vi "GetOuterLoopDataField.vi"(10 "Telemetry Data":string, 11 "Cluster in":refnum<vi>) -> (3 "Array":string[](array[string]))   [LabVIEW 2016]
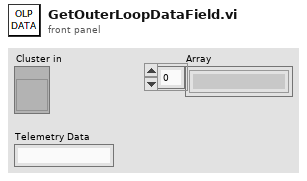
[diagram p1: front panel]
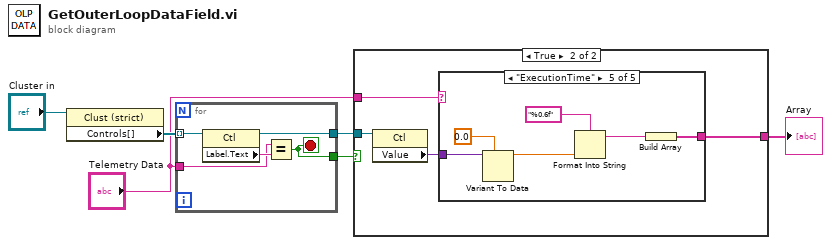
[diagram p0: block diagram]
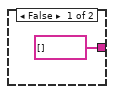
[diagram p2: hidden frame]
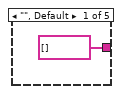
[diagram p3: hidden frame]
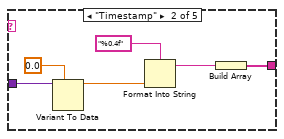
[diagram p4: hidden frame]
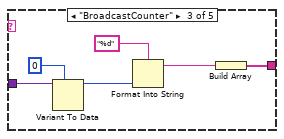
[diagram p5: hidden frame]
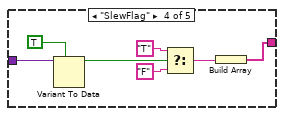
[diagram p6: hidden frame]
diagram:
  n1 = property on="Property Node" class="Clust (strict)"(reference="Cluster in") -> ("Controls[]"=w5:refnum<vi>[])  [unwired: 1 in, 2 out]
  n2 = for {
    tunnel: w5 -> [w11] mode=indexing
    tunnel: [w10] -> w2
    tunnel: "Telemetry Data" -> [w8]
    tunnel: [w7] -> w1
    stop <- w7 stop-if-true
    n3 = property on="Property Node" class="Ctl"(reference=w11) -> (reference out=w10:refnum<vi>, "Label.Text"=w9:string)  [unwired: 1 in, 1 out]
    n4 = Equal?(x=w8, y=w9) -> (x = y?=w7:bool)
  }
  n5 = case shown="True" w1 {
    tunnel: "Telemetry Data" -> [_ w16]
    tunnel: w2 -> [_ w15]
    tunnel: [string[] [] w13] -> w6
    frame False {
    }
    frame True {
      n6 = property on="Property Node" class="Ctl"(reference=w15) -> ("Value"=w14:variant)  [unwired: 1 in, 2 out]
      n7 = case shown="\"ExecutionTime\"" w16 {
        tunnel: [string[] [] w21 w27 w32 w40] -> w13
        tunnel: w14 -> [_ w19 w25 w36 w38]
        frame "", Default {
        }
        frame "Timestamp" {
          n8 = Variant To Data(type=0.0, Variant=w19) -> (data=w20:dbl)  [unwired: 1 in, 1 out]
          n9 = Format Into String(format string="%0.4f", w20) -> (resulting string=w22:string)  [unwired: 2 in, 1 out]
          n10 = Build Array(w22) -> (w21:string[])
        }
        frame "BroadcastCounter" {
          n11 = Variant To Data(type=i16 0, Variant=w25) -> (data=w26:i16)  [unwired: 1 in, 1 out]
          n12 = Format Into String(format string="%d", w26) -> (resulting string=w28:string)  [unwired: 2 in, 1 out]
          n13 = Build Array(w28) -> (w27:string[])
        }
        frame "SlewFlag" {
          n14 = Variant To Data(type=TRUE, Variant=w36) -> (data=w34:bool)  [unwired: 1 in, 1 out]
          n15 = Select(t="T", s=w34, f="F") -> (s? t:f=w33:string)
          n16 = Build Array(w33) -> (w32:string[])
        }
        frame "ExecutionTime" {
          n17 = Variant To Data(type=sgl 0.0, Variant=w38) -> (data=w39:sgl)  [unwired: 1 in, 1 out]
          n18 = Format Into String(format string="%0.6f", w39) -> (resulting string=w41:string)  [unwired: 2 in, 1 out]
          n19 = Build Array(w41) -> (w40:string[])
        }
      }
    }
  }
  "Array" <- w6
